vi "SVM_Train_FromFile_Simple.vi"(8 "error in (no error)":errorcluster) -> (0 "error out":errorcluster, 3 "Binary Confusion Matrix":T1)   [LabVIEW 2014]
uses:
  Controls/Kernel.ctl
  Libsvm Wrapper/Controls/svm_kernel_type.ctl
  Controls/Parameters C_SVC.ctl
  Controls/Options Training.ctl
  Tools/Controls/Binary_ConfusionMatrix.ctl
  SubVIs/SVM Train C_SVC.vi
  Libsvm Wrapper/svm_train.vi
panel:
  in  "Options":T2={"cache_size"=200.0, "eps"=0.001, "shrinking"=TRUE, "probability"=FALSE}
  in  "Param C_SVC":T3={"C"=1.0, "weight_label"=[], "weight"=[]}
  in  "Kernel":T4
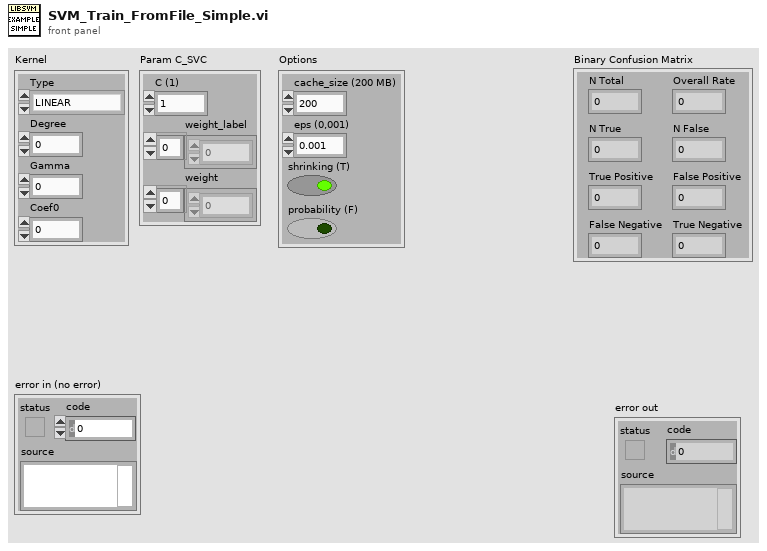
[diagram p1: front panel]
types:
  T1 = typedef "Binary_ConfusionMatrix.ctl" = cluster{"N Total":u32, "N True":u32, "N False":u32, "Overall Rate":dbl, "True Positive":dbl, "False Positive":dbl, "False Negative":dbl, "True Negative":dbl}
  T2 = typedef "Options Training.ctl" = cluster{"cache_size":dbl, "eps":dbl, "shrinking":bool, "probability":bool}
  T3 = typedef "Parameters C_SVC.ctl" = cluster{"C":dbl, "weight_label":i32[], "weight":dbl[]}
  T4 = typedef "Kernel.ctl" = cluster{"Type":T5, "Degree":i32, "Gamma":dbl, "Coef0":dbl}
  T5 = typedef "svm_kernel_type.ctl" = enum32{"LINEAR", "POLY", "RBF", "SIGMOID", "PRECOMPUTED"}
  T6 = cluster{"X lower":dbl, "X upper":dbl, "Y lower":dbl, "Y upper":dbl}
  T7 = typedef "svm_problem.ctl" = cluster{"y":dbl[], "x":cluster{T8[]}[]}
  T8 = typedef "svm_node.ctl" = cluster{"index":i32, "value":dbl}
  T9 = typedef "svm_model.ctl" = cluster{"param":T10, "nr_class":i32, "l":i32, "SV":cluster{"Array":T8[]}[], "sv_coef":dbl[][], "rho":dbl[], "probA":dbl[], "probB":dbl[], "sv_indices":i32[], "label":i32[], "nSV":i32[]}
  T10 = typedef "svm_parameter.ctl" = cluster{"svm_type":T11, "kernel_type":T5, "degree":i32, "gamma":dbl, "coef0":dbl, "cache_size":dbl, "eps":dbl, "C":dbl, "weight_label":i32[], "weight":dbl[], "nu":dbl, "p":dbl, "shrinking":bool, "probability":bool}
  T11 = typedef "svm_type.ctl" = enum32{"C_SVC", "NU_SVC", "ONE_CLASS", "EPSILON_SVR", "NU_SVR"}
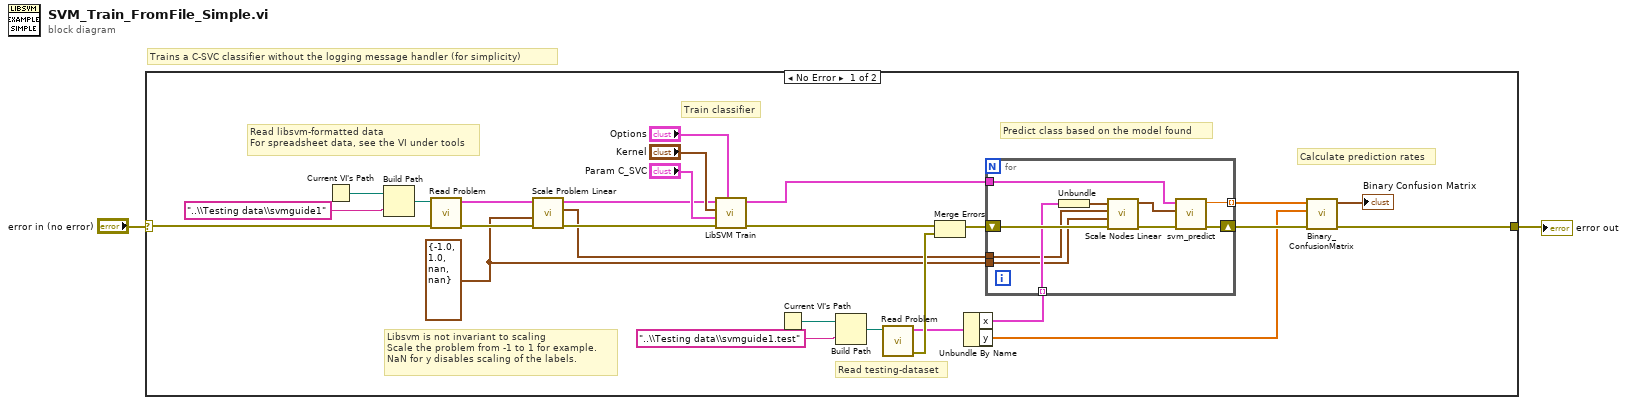
[diagram p0: block diagram]
diagram:
  # "Trains a C-SVC classifier without the logging message handler (for simplicity)"
  n1 = case shown="No Error" "error in (no error)" {
    selector: "error in (no error)" -> [w26 w40]
    tunnel: [w5 w40] -> w2
    frame No Error {
      w9 = T6 {"X lower"=-1.0, "X upper"=1.0, "Y lower"=nan, "Y upper"=nan} ("Scaling limits")
      # "Calculate prediction rates"
      # "Predict class based on the model found"
      # "Train classifier"
      # "Read testing-dataset"
      # "Libsvm is not invariant to scaling\nScale the problem from -1 to 1 for example.\nNaN for y disables scaling of the labels."
      # "Read libsvm-formatted data\nFor spreadsheet data, see the VI under tools"
      n2 = Current VI's Path() -> (path=w27:path)
      n3 = Build Path(base path=w27, name or relative path="..\\Testing data\\svmguide1") -> (appended path=w29:path)
      n4 = call "Read Problem.vi"("error in (no error)"=w26, "file path (use dialog)"=w29) -> ("error out"=w22:errorcluster, "svm_problem"=w21:T7)  [unwired: 8 in]
      n5 = call "Scale Problem Linear.vi"("error in (no error)"=w22, "Scaling limits"=w9, "Problem"=w21) -> ("error out"=w19:errorcluster, "xmaxmin"=w10:cluster{"min":dbl, "max":dbl}[], "Scaled problem"=w20:T7)  [unwired: 5 in, 1 out]
      n6 = call-poly "LibSVM Train.vi"("Options"="Options", "error in (no error)"=w19, "Param C_SVC"="Param C_SVC", "Kernel"="Kernel", "Problem"=w20) -> ("error out"=w15:errorcluster, "Model"=w8:T9)  [unwired: 5 in]
      n7 = Current VI's Path() -> (path=w16:path)
      n8 = Build Path(base path=w16, name or relative path="..\\Testing data\\svmguide1.test") -> (appended path=w18:path)
      n9 = call "Read Problem.vi"("file path (use dialog)"=w18) -> ("error out"=w14:errorcluster, "svm_problem"=w12:T7)  [unwired: 9 in]
      n10 = Merge Errors(w15, w14) -> (w13:errorcluster)
      n11 = Unbundle By Name(w12) -> ("x"=w11:cluster{T8[]}[], "y"=w4:dbl[])
      n12 = for {
        shift-right: [w33] -> w6
        shift-left: w13 -> [w39]
        tunnel: w11 -> [w38] mode=indexing
        tunnel: w10 -> [w36]
        tunnel: w9 -> [w35]
        tunnel: w8 -> [w34]
        tunnel: [w30] -> w7 mode=indexing
        n13 = Unbundle(w38) -> (w37:T8[])
        n14 = call "Scale Nodes Linear.vi"("error in (no error)"=w39, "Scaling limits"=w35, "xminmax"=w36, "x"=w37) -> ("error out"=w32:errorcluster, "x scaled"=w31:T8[])  [unwired: 6 in]
        n15 = call "svm_predict.vi"("error in (no error)"=w32, "X"=w31, "Model"=w34) -> ("error out"=w33:errorcluster, "Predicted label"=w30:dbl)  [unwired: 7 in]
      }
      n16 = call "Binary_ConfusionMatrix.vi"("error in (no error)"=w6, "Actual Labels"=w4, "Predicted Labels"=w7) -> ("error out"=w5:errorcluster, "Binary Confusion Matrix"=→"Binary Confusion Matrix":T1)  [unwired: 7 in]
    }
    frame Error {
    }
  }
  "error out" <- w2
